vi "splash.vi"() -> ()   [LabVIEW 2022 SP3]
panel:
  out "notification":string
  # "Splash Screen"
  # "Run me.  Notifications\nappear below."
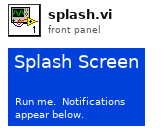
[diagram p1: front panel]
types:
  T1 = enum32{"Invalid", "Standard", "Closed", "Hidden", "Minimized", "Maximized"}
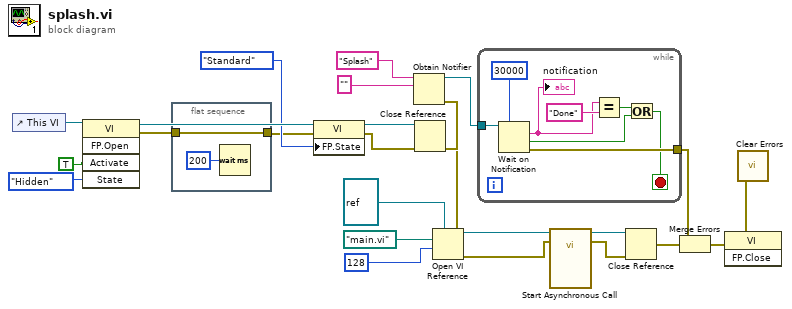
[diagram p0: block diagram]
diagram:
  n1 = control-ref of="This VI"() -> (w13:refnum<vi>)
  n2 = invoke class="VI" method="FP.Open"(reference=w13, "Activate"=TRUE ("Activate?"), "State"=T1."Hidden") -> (reference out=w11:refnum<vi>, error out=w12:errorcluster)  [unwired: 2 in, 3 out]
  n3 = flat-sequence {
    tunnel: [w26] -> w9
    tunnel: w12 -> [w26]
    frame #0 {
      n4 = Wait (ms)(milliseconds to wait=u32 200) -> ()  [unwired: 1 out]
    }
  }
  n5 = property class="VI"(reference=w11, error in=w9, "FP.State"=T1."Standard" ("Front Panel Window:State")) -> (reference out=w8:refnum<vi>, error out=w7:errorcluster)
  n6 = Close Reference(reference=w8, error in (no error)=w7) -> (error out=w6:errorcluster)
  n7 = Obtain Notifier(name (unnamed)="Splash", notification data type="", error in (no error)=w6) -> (notifier out=w5:refnum<notifier>, error out=w4:errorcluster)  [unwired: 1 in, 1 out]
  n8 = Open VI Reference(type specifier VI Refnum (for type only)=refnum<vi> refnum, vi path=path "main.vi", options=128, error in (no error)=w4) -> (vi reference=w2:refnum<vi>, error out=w18:errorcluster)  [unwired: 2 in]
  n9 = while {
    tunnel: w5 -> [w35]
    tunnel: [w32] -> w25
    stop <- w31 stop-if-true
    n10 = Wait on Notification(notifier=w35, timeout in ms (-1)=30000) -> (notification=w28:string, timed out?=w29:bool, error out=w32:errorcluster)  [unwired: 2 in, 1 out]
    "notification" <- w28
    n11 = Equal?(x=w28, y="Done") -> (x = y?=w30:bool)
    n12 = Or(x=w30, y=w29) -> (x .or. y?=w31:bool)
  }
  n13 = call-by-ref "Start Asynchronous Call"(reference=w2, error in=w18) -> (reference out=w3:refnum<vi>, error out=w22:errorcluster)  [unwired: 12 in]
  n14 = Close Reference(reference=w3, error in (no error)=w22) -> (error out=w21:errorcluster)
  n15 = Merge Errors(w25, w21) -> (w24:errorcluster)
  n16 = invoke class="VI" method="FP.Close"(error in=w24) -> (error out=w16:errorcluster)  [unwired: 2 in, 2 out]
  n17 = call <vilib>:"Clear Errors.vi"("error in (no error)"=w16) -> ()  [unwired: 5 in, 2 out]
